vi "Destroy.vi"(0 "reference":refnum<class "BentStyle.lvclass">, 5 "error in (no error)":errorcluster) -> (19 "error out":errorcluster)   [LabVIEW 2020, in "BentStyle.lvclass"]
doc: "Destroys an object created with a BentStyle constructor VI or a subclass of the BentStyle class. This VI must be reentrant.\n\n[GOOP 2.1]"
uses:
  <resource>/Framework/Providers/Open_GDS/UML/BentStyle_class/BentStyle.lvclass
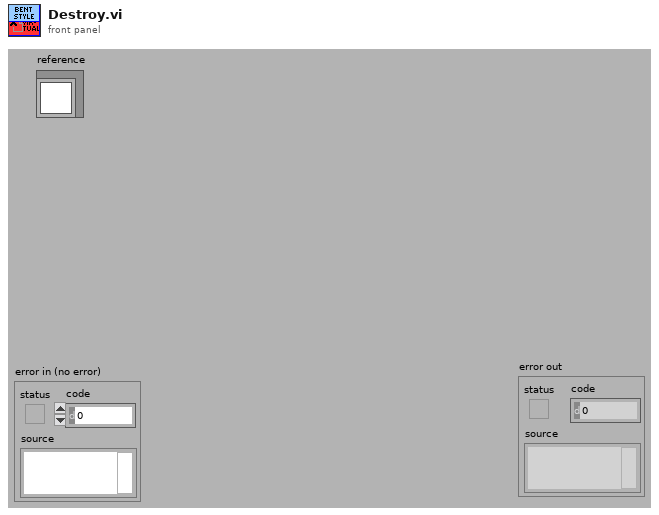
[diagram p1: front panel]
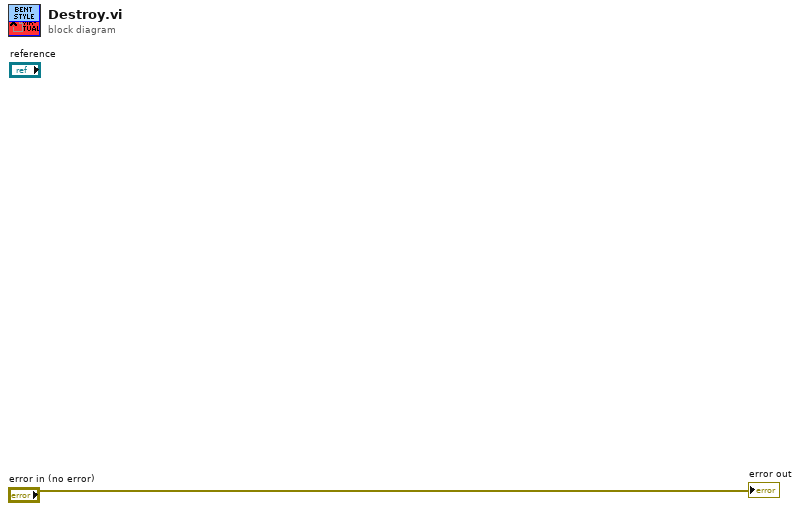
[diagram p0: block diagram]
diagram:
  "error out" <- "error in (no error)"
